vi "getBounds.vi"(0 "reference":refnum<class "MultiLineString.lvclass">, 1 "graphics":refnum<class "Graphics.lvclass">, 5 "error in (no error)":errorcluster) -> (14 "reference out":refnum<class "MultiLineString.lvclass">, 15 "bounds":T1 {"height" format="%.2f"; "width" format="%.2f"; "y" format="%.2f"; "x" format="%.2f"}, 19 "error out":errorcluster)   [LabVIEW 2016, in "MultiLineString.lvclass"]
doc: "public Rectangle2D getBounds(Graphics2D g2)"
uses:
  <resource>/Framework/Providers/Open_GDS/UML/MultiLineString_class/MultiLineString.lvclass
  <resource>/Framework/Providers/Open_GDS/UML/General/Rectangle/Rectangle Rectangle2D.ctl
  <resource>/Framework/Providers/Open_GDS/UML/Graphics_class/Graphics.lvclass
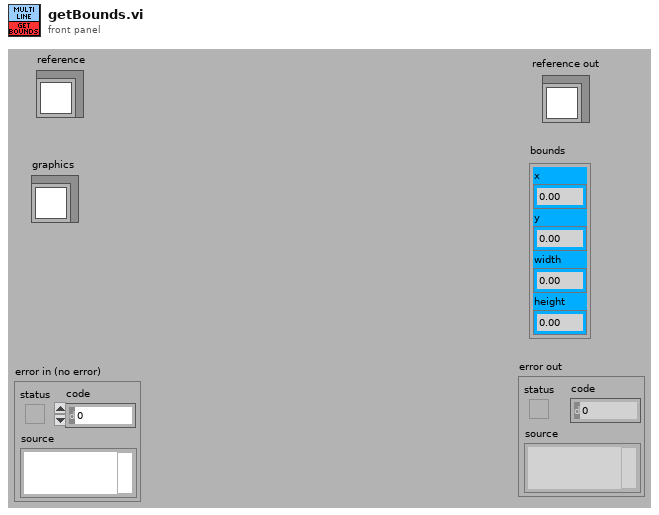
[diagram p1: front panel]
types:
  T1 = typedef "Rectangle Rectangle2D.ctl" = cluster{"x":dbl, "y":dbl, "width":dbl, "height":dbl}
  T2 = typedef "MultiLineString.lvclass/ObjectAttributes.ctl" = cluster{"GAP":i32, "text":string, "justification":T3, "size":T4, "underlined":bool}
  T3 = typedef "MultiLineString.lvclass/JustificationType.ctl" = enum16{"LEFT", "CENTER", "RIGHT"}
  T4 = typedef "MultiLineString.lvclass/SizeType.ctl" = enum16{"LARGE", "NORMAL", "SMALL"}
  T5 = typedef "Graphics.lvclass/LvFontType.ctl" = enum16{"User-specified Font", "Application Font", "System Font", "Dialog Font"}
  T6 = typedef "Graphics.lvclass/FontType.ctl" = cluster{"Font Name:":string, "Size":i16, "Strikeout?":bool, "Italic?":bool, "Underline?":bool, "Outline?":bool, "Shadow?":bool, "Bold?":bool}
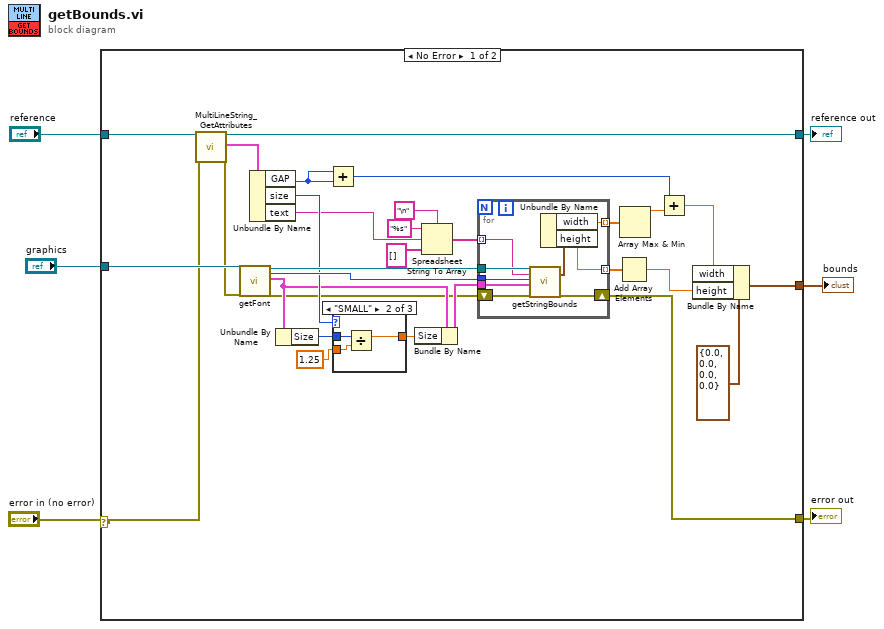
[diagram p0: block diagram]
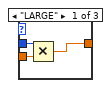
[diagram p2: hidden frame]
diagram:
  n1 = case shown="No Error" "error in (no error)" {
    selector: "error in (no error)" -> [w31 w53]
    tunnel: "reference" -> [w36 w54]
    tunnel: [w35 w53] -> w5
    tunnel: [w34 w54] -> w4
    tunnel: [w33 _] -> w2
    tunnel: "graphics" -> [w32 _]
    frame No Error {
      n2 = call <resource>:"MultiLineString_GetAttributes.vi"("reference in"=w36, "error in (no error)"=w31) -> ("reference out"=w34:refnum<class "MultiLineString.lvclass">, "Data"=w7:T2, "error out"=w8:errorcluster)  [unwired: 1 in, 14 out]
      n3 = call <resource>:"getFont.vi"("reference"=w32, "error in (no error)"=w8) -> ("reference out"=w30:refnum<class "Graphics.lvclass">, "fontType"=w29:T5, "font"=w25:T6, "error out"=w12:errorcluster)  [unwired: 14 out]
      n4 = Unbundle By Name(w7) -> ("GAP"=w17:i32, "size"=w26:T4, "text"=w19:string)
      n5 = Unbundle By Name(w25) -> ("Size"=w28:i16)
      n6 = Add(x=w17, y=w17) -> (x+y=w14:i32)
      n7 = case shown="\"SMALL\"" w26 {
        tunnel: w28 -> [w48 w50 w52]
        tunnel: 1.25 ("y") -> [w47 w51 _]
        tunnel: [w46 w49 w52] -> w23
        frame "LARGE" {
          n8 = Multiply(x=w48, y=w47) -> (x*y=w46:dbl)
        }
        frame "SMALL" {
          n9 = Divide(x=w50, y=w51) -> (x/y=w49:dbl)
        }
        frame "NORMAL", Default {
        }
      }
      n10 = Bundle By Name(cluster=w25, "Size"=w23) -> (w24:T6)
      n11 = Spreadsheet String To Array(delimiter (Tab)="\n", format string="%s", spreadsheet string=w19, array type (2D Dbl)=string[] []) -> (array=w18:string[])
      n12 = for {
        tunnel: w30 -> [w45]
        tunnel: w29 -> [w44]
        tunnel: w24 -> [w43]
        tunnel: w18 -> [w42] mode=indexing
        tunnel: [w40] -> w16 mode=indexing
        tunnel: [w39] -> w13 mode=indexing
        shift-right: [w37] -> w35
        shift-left: w12 -> [w38]
        n13 = call-dynamic "getStringBounds.vi"("reference"=w45, "text"=w42, "fontType"=w44, "font"=w43, "error in (no error)"=w38) -> ("bounds"=w41:T1, "error out"=w37:errorcluster)  [unwired: 13 out]
        n14 = Unbundle By Name(w41) -> ("width"=w40:dbl, "height"=w39:dbl)
      }
      n15 = Add Array Elements(numeric array=w13) -> (sum=w9:dbl)
      n16 = Array Max & Min(array=w16) -> (max value=w15:dbl)  [unwired: 3 out]
      n17 = Add(x=w14, y=w15) -> (x+y=w10:dbl)
      n18 = Bundle By Name(cluster=T1 {"x"=0.0, "y"=0.0, "width"=0.0, "height"=0.0} ("bounds"), "width"=w10, "height"=w9) -> (w33:T1)
    }
    frame Error {
    }
  }
  "reference out" <- w4
  "error out" <- w5
  "bounds" <- w2
